vi "Init.vi"(8 "error in (no error)":errorcluster, 10 "Instrument String":variant, 11 "Tektronix Scope in":refnum<class "Tektronix MSO5.lvclass">) -> (0 "error out":errorcluster, 2 "Found?":bool=TRUE, 3 "Tektronix Scope out":refnum<class "Tektronix MSO5.lvclass">)   [LabVIEW 2025, in "Scope.lvlib" / "Tektronix MSO5.lvclass"]
uses:
  Tektronix MSO5.lvclass
  C:/Working copy/tss/Plugin/Engines/Scope/Scope Instrument/Scope Instrument.lvclass
  Scope configuration/Scope configuration.lvclass
  C:/Users/Public/Documents/Sandia National Labs/TSS Plugin/Abstract Engine.lvlibp/Plugin/Abstract/Instrument configuration/Instrument configuration.lvclass
  Tektronix MSO5.lvclass/Tektronix MSO5.ctl
  Users/Public/Documents/Sandia National Labs/TSS Plugin/Abstract Engine.lvlibp/Plugin/Abstract/Instrument configuration/Read Instrument Setting.vi
  Users/Public/Documents/Sandia National Labs/TSS Plugin/CEF.lvlibp/serializable configuration/CEF_serializable configuration.lvclass
  <instrlib>/Tektronix MSO5 Series/Utilities/MS058LP Library.lvlib
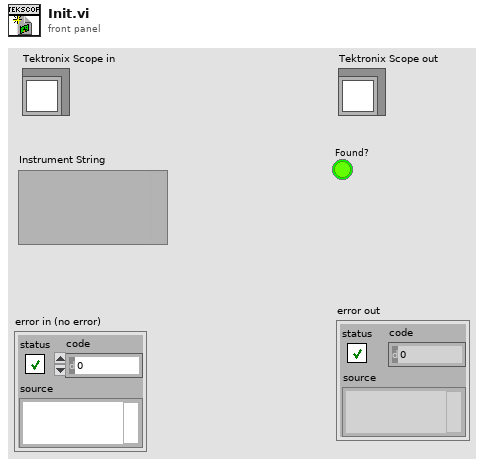
[diagram p1: front panel]
types:
  T1 = typedef "Abstract Engine.lvlibp/Instrument configuration.lvclass/Default Instrument.ctl" = cluster{"Type":string, "Address":string, "SW Alias":string, "Description":string, "Enabled":bool}
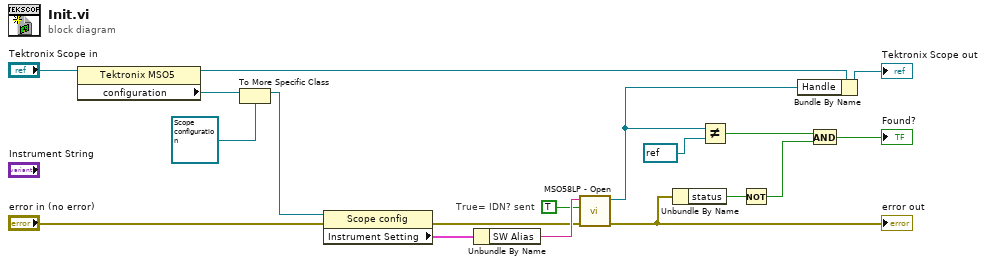
[diagram p0: block diagram]
diagram:
  # "True= IDN? sent"
  n1 = property class="Tektronix MSO5"(reference="Tektronix Scope in") -> (reference out=w15:refnum<class "Tektronix MSO5.lvclass">, "configuration"=w14:refnum<class "CEF_serializable configuration.lvclass">)  [unwired: 1 in, 1 out]
  n2 = To More Specific Class(target class=refnum<class "Scope configuration.lvclass"> refnum ("Scope.lvlib:Scope configuration.lvclass"), reference=w14) -> (specific class reference=w13:refnum<class "Scope configuration.lvclass">)  [unwired: 1 in, 1 out]
  n3 = property class="Scope config"(reference=w13, error in="error in (no error)") -> (error out=w1:errorcluster, "Instrument Setting"=w16:T1)  [unwired: 1 out]
  n4 = Unbundle By Name(w16) -> ("SW Alias"=w12:string)
  n5 = call <instrlib>:"MSO58LP - Open.vi"("error in"=w1, "ID Query (True)"=TRUE, "VISA In"=w12) -> ("error out"=w6:errorcluster, "VISA Out"=w4:refnum<visa-resource-name>)  [unwired: 7 in]
  "error out" <- w6
  n6 = Unbundle By Name(w6) -> ("status"=w8:bool)
  n7 = Not Equal?(x=w4, y=refnum<visa-resource-name> refnum ("VISA Out")) -> (x != y?=w7:bool)
  n8 = Not(x=w8) -> (.not. x?=w9:bool)
  n9 = Bundle By Name(cluster=w15, "Handle"=w4) -> (→"Tektronix Scope out":refnum<class "Tektronix MSO5.lvclass">)
  n10 = And(x=w7, y=w9) -> (x .and. y?=→"Found?":bool)
